vi "Close.vi"(8 "error in (no error)":errorcluster, 11 "Instrument in":refnum<class "Instrument.lvclass">) -> (0 "error out":errorcluster, 3 "Instrument out":refnum<class "Instrument.lvclass">)   [LabVIEW 2019, in "Instrument.lvlib" / "Instrument.lvclass"]
doc: "Closes a remote connection to an Instrument instance. This can be called on its own or is called automatically by \"Remote Client.vim\""
uses:
  Instrument.lvclass
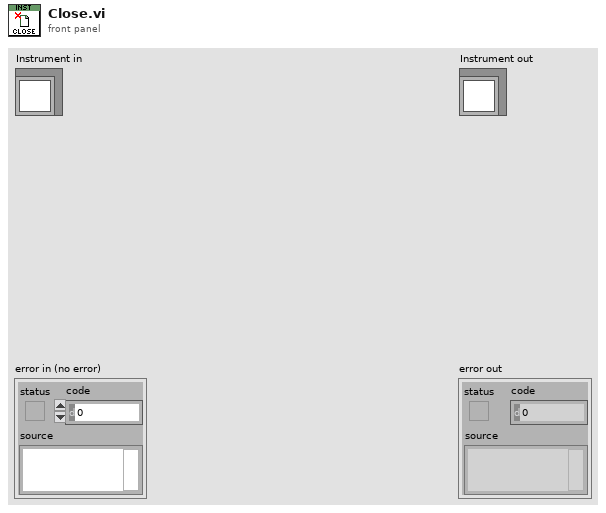
[diagram p1: front panel]
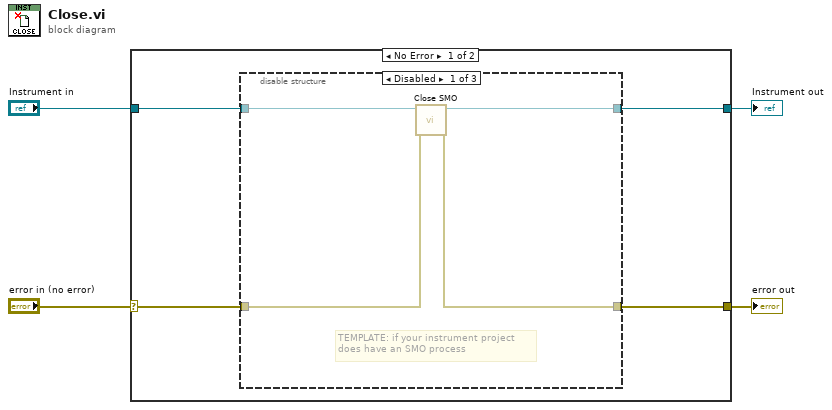
[diagram p0: block diagram]
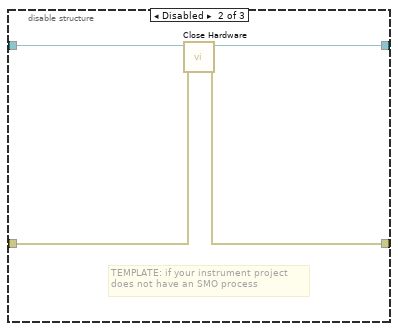
[diagram p2: hidden frame]
diagram:
  n1 = case shown="No Error" "error in (no error)" {
    selector: "error in (no error)" -> [w6 w20]
    tunnel: [w5 w20] -> w3
    tunnel: [w8 w19] -> w1
    tunnel: "Instrument in" -> [w7 w19]
    frame No Error {
      n2 = disable-structure shown="Disabled" {
        disable-tunnel: [w12 w15 w18] -> w8
        disable-tunnel: w7 -> [w11 w16 w18]
        disable-tunnel: w6 -> [w10 w14 w17]
        disable-tunnel: [w9 w13 w17] -> w5
        frame Disabled {
          # "TEMPLATE: if your instrument project\ndoes have an SMO process"
          n3 = call "Close SMO.vi"("error in (no error)"=w10, "Instrument in"=w11) -> ("error out"=w9:errorcluster, "Instrument out"=w12:refnum<class "Instrument.lvclass">)  [unwired: 8 in]
        }
        frame Disabled {
          # "TEMPLATE: if your instrument project\ndoes not have an SMO process"
          n4 = call-dynamic "Close Hardware.vi"("error in (no error)"=w14, "Instrument in"=w16) -> ("error out"=w13:errorcluster, "Instrument out"=w15:refnum<class "Instrument.lvclass">)  [unwired: 8 in]
        }
        frame Enabled {
        }
      }
    }
    frame Error {
    }
  }
  "error out" <- w3
  "Instrument out" <- w1
